vi "add filename if missing.vi"(10 "remote path (relative to root)":path, 11 "local path":path) -> (3 "appended path":path)   [LabVIEW 2013, in "PL Framework Configuration Tool.lvlib"]
uses:
  PL Framework Configuration Tool.lvlib
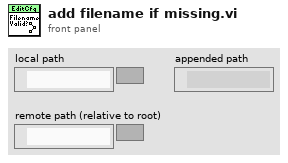
[diagram p1: front panel]
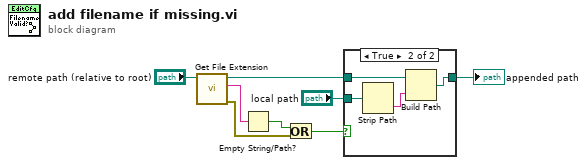
[diagram p0: block diagram]
diagram:
  n1 = call <vilib>:"Get File Extension.vi"("file"="remote path (relative to root)") -> ("error out"=w2:errorcluster, "lowercase file extension"=w3:string, "dup file"=w7:path)  [unwired: 7 in, 1 out]
  n2 = Empty String/Path?(string/path=w3) -> (empty?=w4:bool)
  n3 = Or(x=w4, y=w2) -> (x .or. y?=w5:bool)
  n4 = case shown="True" w5 {
    tunnel: "local path" -> [_ w13]
    tunnel: w7 -> [w9 w11]
    tunnel: [w9 w10] -> w8
    frame False {
    }
    frame True {
      n5 = Strip Path(path=w13) -> (name=w12:string)  [unwired: 1 out]
      n6 = Build Path(base path=w11, name or relative path=w12) -> (appended path=w10:path)
    }
  }
  "appended path" <- w8
